vi "Read AutoAge_ini.vi"(12 "AutoAge.ini File Path":path=path "\\\\Beco\\autoage/config/autoage.ini") -> (0 "Client ini File Path":path, 1 "Failing File Path":path, 2 "Early File Path":path, 3 "Equation File Path":path, 4 "Aging Macros File Path":path, 5 "Func Start File Path":path, 6 "Crystal Archive File Path":path, 7 "Func File Path":path, 8 "Archive File Path":path, 9 "SharePointTransferPath":path, 10 "OldData File Path":path, 11 "Passing File Path":path, 13 "ID File Path":path, 14 "Run File Path":path, 15 "Data File Path":path)   [LabVIEW 2021]
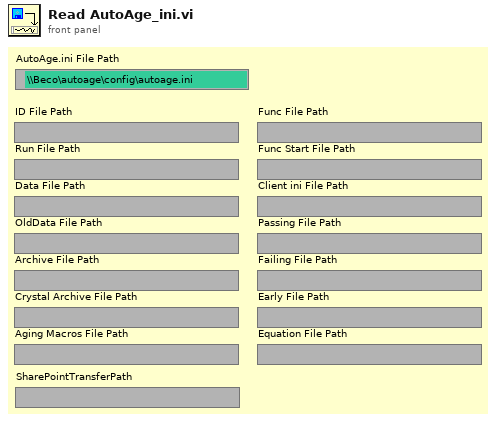
[diagram p1: front panel]
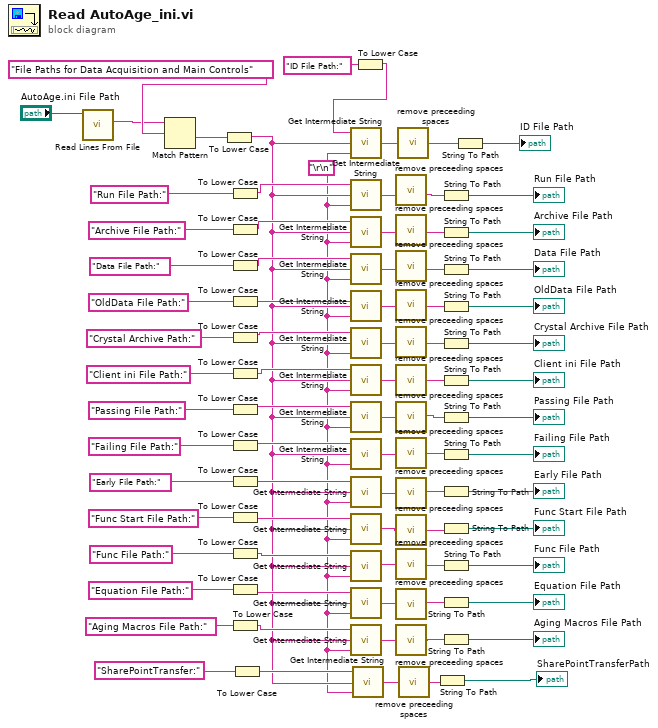
[diagram p0: block diagram]
diagram:
  w4 = "\r\n"
  n1 = call <vilib>:"Read Lines From File.vi"("file path (dialog if empty)"="AutoAge.ini File Path") -> ("line string"=w79:string)  [unwired: 5 in, 3 out]
  n2 = Match Pattern(string=w79, regular expression="File Paths for Data Acquisition and Main Controls") -> (after substring=w76:string)  [unwired: 1 in, 3 out]
  n3 = To Lower Case(string=w76) -> (all lower case string=w5:string)
  n4 = To Lower Case(string="Run File Path:") -> (all lower case string=w50:string)
  n5 = To Lower Case(string="Archive File Path:") -> (all lower case string=w51:string)
  n6 = To Lower Case(string="Data File Path:") -> (all lower case string=w52:string)
  n7 = To Lower Case(string="OldData File Path:") -> (all lower case string=w53:string)
  n8 = To Lower Case(string="Crystal Archive Path:") -> (all lower case string=w54:string)
  n9 = To Lower Case(string="Client ini File Path:") -> (all lower case string=w55:string)
  n10 = To Lower Case(string="Passing File Path:") -> (all lower case string=w56:string)
  n11 = To Lower Case(string="Failing File Path:") -> (all lower case string=w57:string)
  n12 = To Lower Case(string="Early File Path:") -> (all lower case string=w58:string)
  n13 = To Lower Case(string="Func Start File Path:") -> (all lower case string=w59:string)
  n14 = To Lower Case(string="Func File Path:") -> (all lower case string=w60:string)
  n15 = To Lower Case(string="Equation File Path:") -> (all lower case string=w61:string)
  n16 = To Lower Case(string="Aging Macros File Path:") -> (all lower case string=w62:string)
  n17 = To Lower Case(string="SharePointTransfer:") -> (all lower case string=w6:string)
  n18 = call "Get Intermediate String.vi"("End Delimiter"=w4, "Input String"=w5, "Start Delimiter"=w50) -> ("Output String"=w33:string)
  n19 = call "Get Intermediate String.vi"("End Delimiter"=w4, "Input String"=w5, "Start Delimiter"=w51) -> ("Output String"=w32:string)
  n20 = call "Get Intermediate String.vi"("End Delimiter"=w4, "Input String"=w5, "Start Delimiter"=w52) -> ("Output String"=w31:string)
  n21 = call "Get Intermediate String.vi"("End Delimiter"=w4, "Input String"=w5, "Start Delimiter"=w53) -> ("Output String"=w30:string)
  n22 = call "Get Intermediate String.vi"("End Delimiter"=w4, "Input String"=w5, "Start Delimiter"=w54) -> ("Output String"=w29:string)
  n23 = call "Get Intermediate String.vi"("End Delimiter"=w4, "Input String"=w5, "Start Delimiter"=w55) -> ("Output String"=w28:string)
  n24 = call "Get Intermediate String.vi"("End Delimiter"=w4, "Input String"=w5, "Start Delimiter"=w56) -> ("Output String"=w27:string)
  n25 = call "Get Intermediate String.vi"("End Delimiter"=w4, "Input String"=w5, "Start Delimiter"=w57) -> ("Output String"=w26:string)
  n26 = call "Get Intermediate String.vi"("End Delimiter"=w4, "Input String"=w5, "Start Delimiter"=w58) -> ("Output String"=w25:string)
  n27 = call "Get Intermediate String.vi"("End Delimiter"=w4, "Input String"=w5, "Start Delimiter"=w59) -> ("Output String"=w24:string)
  n28 = call "Get Intermediate String.vi"("End Delimiter"=w4, "Input String"=w5, "Start Delimiter"=w60) -> ("Output String"=w23:string)
  n29 = call "Get Intermediate String.vi"("End Delimiter"=w4, "Input String"=w5, "Start Delimiter"=w61) -> ("Output String"=w22:string)
  n30 = call "Get Intermediate String.vi"("End Delimiter"=w4, "Input String"=w5, "Start Delimiter"=w62) -> ("Output String"=w21:string)
  n31 = call "Get Intermediate String.vi"("End Delimiter"=w4, "Input String"=w5, "Start Delimiter"=w6) -> ("Output String"=w3:string)
  n32 = To Lower Case(string="ID File Path:") -> (all lower case string=w77:string)
  n33 = call "Get Intermediate String.vi"("End Delimiter"=w4, "Input String"=w5, "Start Delimiter"=w77) -> ("Output String"=w35:string)
  n34 = call "remove preceeding spaces.vi"("Raw String"=w33) -> ("Edited String"=w20:string)
  n35 = call "remove preceeding spaces.vi"("Raw String"=w32) -> ("Edited String"=w19:string)
  n36 = call "remove preceeding spaces.vi"("Raw String"=w31) -> ("Edited String"=w18:string)
  n37 = call "remove preceeding spaces.vi"("Raw String"=w30) -> ("Edited String"=w17:string)
  n38 = call "remove preceeding spaces.vi"("Raw String"=w29) -> ("Edited String"=w16:string)
  n39 = call "remove preceeding spaces.vi"("Raw String"=w28) -> ("Edited String"=w15:string)
  n40 = call "remove preceeding spaces.vi"("Raw String"=w27) -> ("Edited String"=w14:string)
  n41 = call "remove preceeding spaces.vi"("Raw String"=w26) -> ("Edited String"=w13:string)
  n42 = call "remove preceeding spaces.vi"("Raw String"=w25) -> ("Edited String"=w12:string)
  n43 = call "remove preceeding spaces.vi"("Raw String"=w24) -> ("Edited String"=w11:string)
  n44 = call "remove preceeding spaces.vi"("Raw String"=w23) -> ("Edited String"=w10:string)
  n45 = call "remove preceeding spaces.vi"("Raw String"=w22) -> ("Edited String"=w9:string)
  n46 = call "remove preceeding spaces.vi"("Raw String"=w21) -> ("Edited String"=w8:string)
  n47 = call "remove preceeding spaces.vi"("Raw String"=w35) -> ("Edited String"=w34:string)
  n48 = call "remove preceeding spaces.vi"("Raw String"=w3) -> ("Edited String"=w2:string)
  n49 = String To Path(string=w2) -> (path=→"SharePointTransferPath":path)
  n50 = String To Path(string=w20) -> (path=→"Run File Path":path)
  n51 = String To Path(string=w19) -> (path=→"Archive File Path":path)
  n52 = String To Path(string=w18) -> (path=→"Data File Path":path)
  n53 = String To Path(string=w17) -> (path=→"OldData File Path":path)
  n54 = String To Path(string=w16) -> (path=→"Crystal Archive File Path":path)
  n55 = String To Path(string=w15) -> (path=→"Client ini File Path":path)
  n56 = String To Path(string=w14) -> (path=→"Passing File Path":path)
  n57 = String To Path(string=w13) -> (path=→"Failing File Path":path)
  n58 = String To Path(string=w12) -> (path=→"Early File Path":path)
  n59 = String To Path(string=w11) -> (path=→"Func Start File Path":path)
  n60 = String To Path(string=w10) -> (path=→"Func File Path":path)
  n61 = String To Path(string=w9) -> (path=→"Equation File Path":path)
  n62 = String To Path(string=w8) -> (path=→"Aging Macros File Path":path)
  n63 = String To Path(string=w34) -> (path=→"ID File Path":path)
